vi "Create ListImp_Common.vi"(5 "ListImp_Reusable in":refnum<class "ListImp_Common.lvclass">, 8 "error in (no error)":errorcluster, 10 "Initial List":i32[](array[numeric]), 11 "ListImp":refnum<class "ListImp.lvclass">) -> (0 "error out":errorcluster, 3 "ListImp_Reusable out":refnum<class "ListImp_Common.lvclass">)   [LabVIEW 2013, in "ListImp_Common.lvclass"]
uses:
  ListImp_Common.lvclass
  source/LapDog.Collections.Lists/ListImp/ListImp.lvclass
  ListImp_Common.lvclass/ListImp_Common.ctl
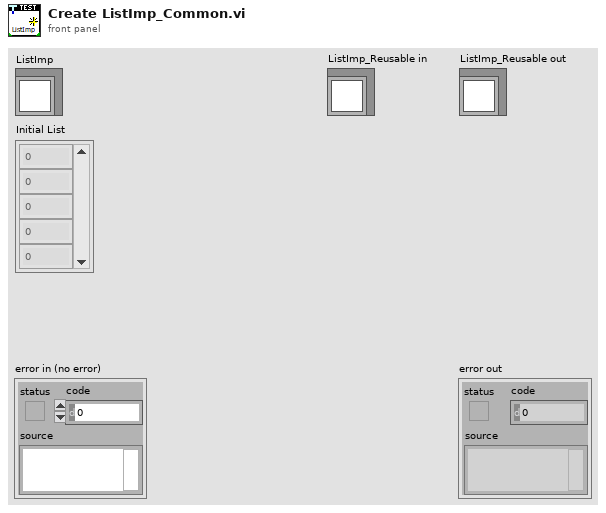
[diagram p1: front panel]
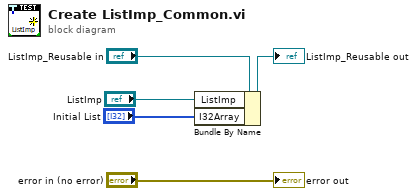
[diagram p0: block diagram]
diagram:
  n1 = Bundle By Name(cluster="ListImp_Reusable in", "ListImp"="ListImp", "I32Array"="Initial List") -> (→"ListImp_Reusable out":refnum<class "ListImp_Common.lvclass">)
  "error out" <- "error in (no error)"
